vi "ATF-Pump-Data Transfer Loop DD.vi"(9 "Data FIFO Ref":T1) -> ()   [LabVIEW 2022 SP3]
uses:
  RT Controls/ATF-Pump-Data FIFO.ctl
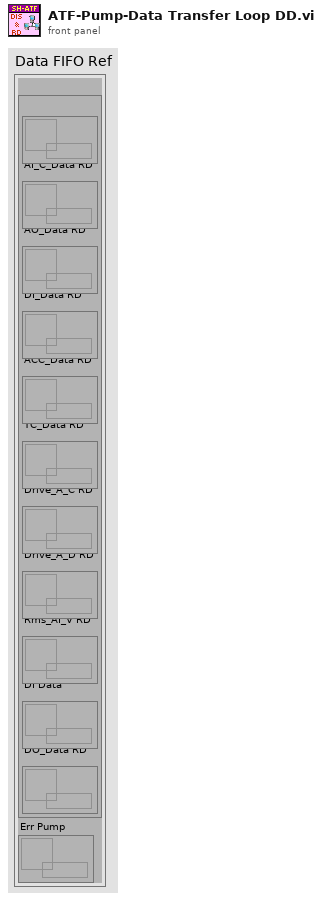
[diagram p1: front panel]
types:
  T1 = typedef "ATF-Pump-Data FIFO.ctl" = cluster{"RD":cluster{"AI_V_Data RD":refnum<queue>, "AI_C_Data RD":refnum<queue>, "AO_Data RD":refnum<queue>, "DI_Data RD":refnum<queue>, "ACC_Data RD":refnum<queue>, "TC_Data RD":refnum<queue>, "Drive_A_C RD":refnum<queue>, "Drive_A_D RD":refnum<queue>, "Rms_AI_V RD":refnum<queue>, "DI Data":refnum<queue>, "DO_Data RD":refnum<queue>}, "Err Pump":refnum<queue>}
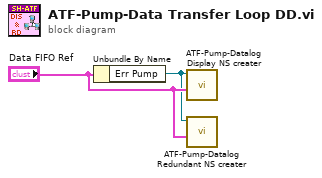
[diagram p0: block diagram]
diagram:
  n1 = Unbundle By Name("Data FIFO Ref") -> ("Err Pump"=w1:refnum<queue>)
  n2 = call "ATF-Pump-Datalog Display NS creater.vi"("Data FIFO Ref"="Data FIFO Ref", "Queue in"=w1) -> ()  [unwired: 10 in]
  n3 = call "ATF-Pump-Datalog Redundant NS creater.vi"("Data FIFO Ref"="Data FIFO Ref", "Queue in"=w1) -> ()  [unwired: 10 in]
